vi "ingest_csv.vi"(4 "optional":T1, 7 "timestampMetadata":refnum<class "timestampMetadata.lvclass">, 8 "error in":errorcluster, 9 "Target":refnum<class "target.lvclass">, 10 "Source":refnum<class "source.lvclass">, 11 "Nominal Client in":refnum<class "Nominal Client.lvclass">) -> (0 "error out":errorcluster, 1 "datasetFileId":string, 2 "datasetRid":string, 3 "Nominal Client out":refnum<class "Nominal Client.lvclass">, 5 "ingestJobRid":string)   [LabVIEW 2020, in "Nominal Client.lvclass"]
doc: "Triggers an ingest job, allowing either creating a new dataset or uploading to an existing one. This endpoint is meant to supersede all other ingestion endpoints as their functionality gets migrated to this one."
uses:
  Nominal Client.lvclass
  datasources/target/target.lvclass
  datasources/source/source.lvclass
  timestampMetadata/timestampMetadata.lvclass
  Nominal Client.lvclass/Nominal Client.ctl
  datasources/target/target.lvclass/target.ctl
  <vilib>/JDP Science/JSONtext/LVClass Serializer/JSONtext LVClass Serializer.lvclass
  nominal types/properties/properties.lvclass
  nominal types/labels/labels.lvclass
  <vilib>/JDP Science/JSONtext/JSONtext.lvlib
  4e81ab5e-e540-474e-8302-0a664eb7b944.vi
  da70c7dd-7914-44ef-86ed-2bc4582d2eab.vi
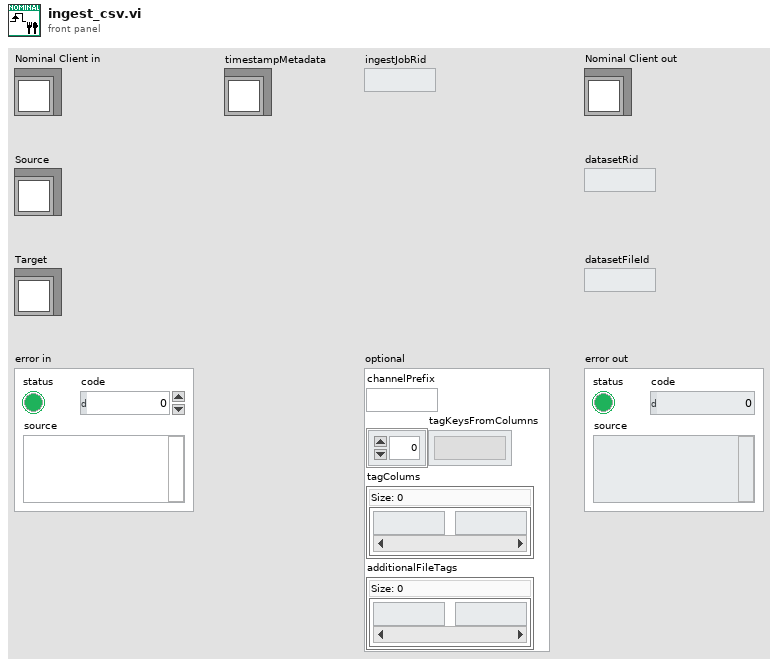
[diagram p1: front panel]
types:
  T1 = cluster{"channelPrefix":string, "tagKeysFromColumns":string[], "tagColums":map{string, string}, "additionalFileTags":map{string, string}}
  T2 = cluster{"details":cluster{"type":string, "dataset":cluster{"datasetFileId":string, "datasetRid":string}}, "ingestJobRid":string}
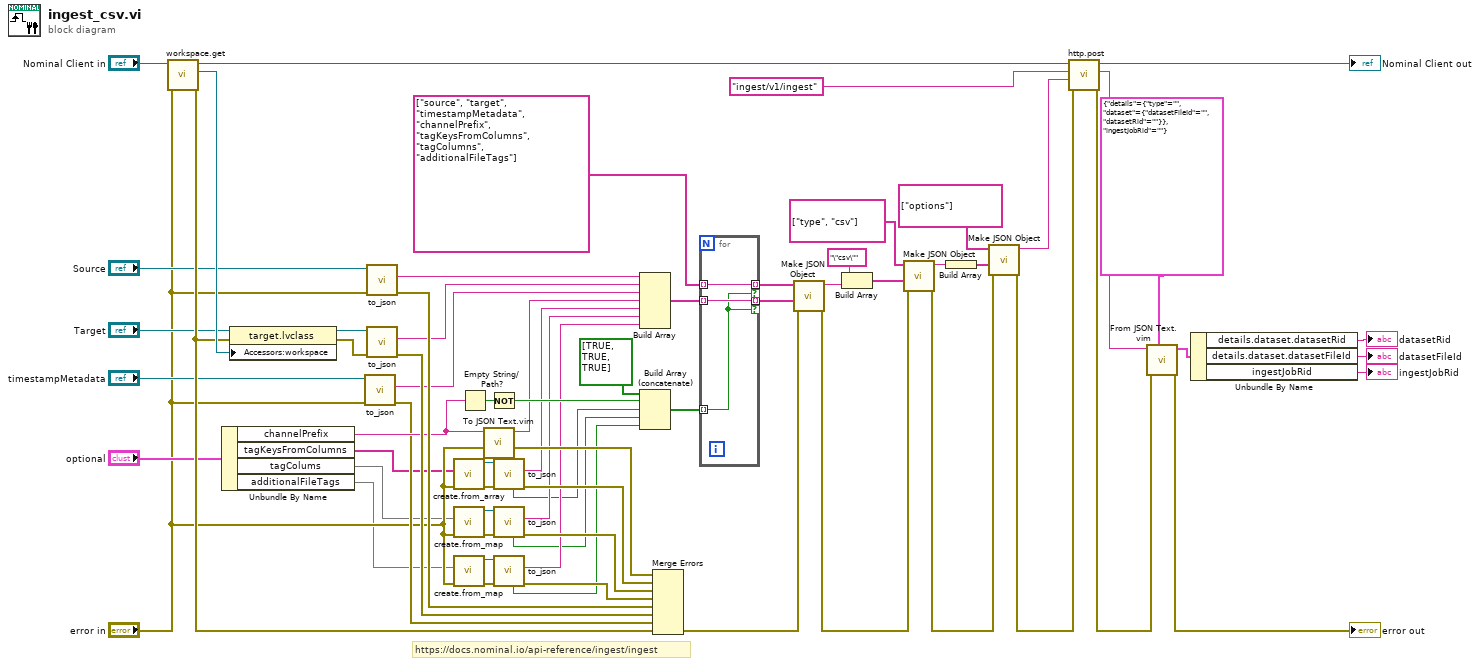
[diagram p0: block diagram]
diagram:
  # "https://docs.nominal.io/api-reference/ingest/ingest"
  n1 = call "workspace.get.vi"("error in"="error in", "Nominal Client in"="Nominal Client in") -> ("error out"=w46:errorcluster, "workspace"=w60:refnum<class "workspace.lvclass">, "Nominal Client out"=w61:refnum<class "Nominal Client.lvclass">)  [unwired: 7 in]
  n2 = Unbundle By Name("optional") -> ("channelPrefix"=w55:string, "tagKeysFromColumns"=w3:string[], "tagColums"=w4:map{string, string}, "additionalFileTags"=w5:map{string, string})
  n3 = property class="target.lvclass"(reference="Target", error in=w46, "Accessors:workspace"=w60) -> (reference out=w63:refnum<class "target.lvclass">, error out=w64:errorcluster)
  n4 = call-dynamic "to_json.vi"("error in"="error in", "timestampMetadata in"="timestampMetadata") -> ("error out"=w45:errorcluster, "json"=w57:string)  [unwired: 6 in, 2 out]
  n5 = call-dynamic "to_json.vi"("error in"="error in", "source in"="Source") -> ("error out"=w66:errorcluster, "json"=w59:string)  [unwired: 6 in, 2 out]
  n6 = call-dynamic "to_json.vi"("error in"=w64, "target in"=w63) -> ("error out"=w65:errorcluster, "json"=w58:string)  [unwired: 6 in, 2 out]
  n7 = call "create.from_array.vi"("error in"="error in", "labels"=w3) -> ("error out"=w7:errorcluster, "labels out"=w8:refnum<class "labels.lvclass">)  [unwired: 8 in]
  n8 = call "create.from_map.vi"("error in"="error in", "properties"=w4) -> ("error out"=w10:errorcluster, "properties out"=w9:refnum<class "properties.lvclass">)  [unwired: 8 in]
  n9 = call "create.from_map.vi"("error in"="error in", "properties"=w5) -> ("error out"=w11:errorcluster, "properties out"=w12:refnum<class "properties.lvclass">)  [unwired: 8 in]
  n10 = Empty String/Path?(string/path=w55) -> (empty?=w56:bool)
  n11 = call "To JSON Text.vim"("error in (no error)"="error in", "Anything"=w55) -> ("error out"=w41:errorcluster, "<JSON>"=w40:string)  [unwired: 8 in]
  n12 = Not(x=w56) -> (.not. x?=w54:bool)
  n13 = call-dynamic "to_json.vi"("error in"=w7, "labels in"=w8) -> ("error out"=w42:errorcluster, "json"=w39:string, "Not Default"=w36:bool)  [unwired: 6 in, 1 out]
  n14 = call-dynamic "to_json.vi"("error in"=w10, "properties in"=w9) -> ("error out"=w43:errorcluster, "json"=w38:string, "Not Default"=w35:bool)  [unwired: 6 in, 1 out]
  n15 = call-dynamic "to_json.vi"("error in"=w11, "properties in"=w12) -> ("error out"=w44:errorcluster, "json"=w37:string, "Not Default"=w34:bool)  [unwired: 6 in, 1 out]
  n16 = Build Array(w59, w58, w57, w40, w39, w38, w37) -> (w52:string[])
  n17 = Build Array (concatenate)(bool[] [TRUE, TRUE, TRUE] ("element"), w54, w36, w35, w34) -> (w48:bool[])
  n18 = Merge Errors(w41, w42, w43, w44, w66, w65, w45, w46) -> (w47:errorcluster)
  n19 = for {
    tunnel: w52 -> [w71] mode=indexing
    tunnel: [w71] -> w51 mode=indexing if=w69
    tunnel: string[] ["source", "target", "timestampMetadata", "channelPrefix", "tagKeysFromColumns", "tagColumns", "additionalFileTags"] ("Item Names") -> [w70] mode=indexing
    tunnel: [w70] -> w49 mode=indexing if=w69
    tunnel: w48 -> [w69] mode=indexing
  }
  n20 = call <vilib>:"Make JSON Object.vi"("error in (no error)"=w47, "JSON Items"=w51, "Item Names"=w49) -> ("error out"=w29:errorcluster, "<JSON>"=w32:string)  [unwired: 7 in]
  n21 = Build Array("\"csv\"" ("JSON"), w32) -> (w31:string[])
  n22 = call <vilib>:"Make JSON Object.vi"("error in (no error)"=w29, "JSON Items"=w31, "Item Names"=string[] ["type", "csv"] ("JSON")) -> ("error out"=w16:errorcluster, "<JSON>"=w18:string)  [unwired: 7 in]
  n23 = Build Array(w18) -> (w19:string[])
  n24 = call <vilib>:"Make JSON Object.vi"("error in (no error)"=w16, "JSON Items"=w19, "Item Names"=string[] ["options"] ("JSON")) -> ("error out"=w15:errorcluster, "<JSON>"=w17:string)  [unwired: 7 in]
  n25 = call "http.post.vi"("error in"=w15, "Request body"=w17, "Path"="ingest/v1/ingest", "Nominal Client in"=w61) -> ("error out"=w22:errorcluster, "Response"=w23:string, "Nominal Client out"=→"Nominal Client out":refnum<class "Nominal Client.lvclass">)  [unwired: 5 in]
  n26 = call "From JSON Text.vim"("Data Type and Default Value"=T2 {"details"={"type"="", "dataset"={"datasetFileId"="", "datasetRid"=""}}, "ingestJobRid"=""}, "error in (no error)"=w22, "JSON"=w23) -> ("error out"=→"error out":errorcluster, "Data out"=w24:T2)  [unwired: 7 in]
  n27 = Unbundle By Name(w24) -> ("details.dataset.datasetRid"=→"datasetRid":string, "details.dataset.datasetFileId"=→"datasetFileId":string, "ingestJobRid"=→"ingestJobRid":string)
